vi "fgv_v-linear_func.vi"() -> (3 "velocity_out":dbl)   [LabVIEW 2019]
uses:
  Ctrl/pid-in-params.ctl
  Ctrl/agv_cmd_v.ctl
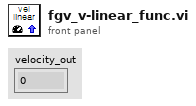
[diagram p1: front panel]
types:
  T1 = typedef "pid-in-params.ctl" = enum16{"read", "write"}
  T2 = cluster{" turn angular speed":dbl, "move linear speed":dbl, "decrease factor linear speed":dbl, "adjust angle margin":dbl}
  T3 = cluster{"deg_agv-lookahead":dbl, "deg_waypoint":dbl, "deg_gap":dbl, "deg_target":dbl, "pid output":dbl, "dis-gap":dbl, "deg_agv-center":dbl}
  T4 = typedef "system_hw.ctl" = cluster{"AGV":enum16{"none", "ERP42", "ERP42mini", "Scout", "Ycar"}, "Lidar 1":enum16{"none", "VLP16", "TIM571", "RPLidar A2", "RPLidar A3"}, "Lidar 2":enum16{"none", "VLP16", "TIM571", "RPLidar A2", "RPLidar A3"}, "GPS":enum16{"none", "F9P", "M8P", "PwrPak7", "19X HVS"}, "Camera":enum16{"none", "C920", "C922", "GT1290C", "MS LifeCam"}, "Joystick":enum16{"none", "joystick"}, "sound":enum16{"none", "speaker"}, "IMU":enum16{"none", "MW-AHRSv1"}}
  T5 = enum16{"none", "ERP42", "ERP42mini", "Scout", "Ycar"}
  T6 = typedef "agv_cmd_v.ctl" = enum16{"write limit", "init stop", "write", "read"}
  T7 = cluster{"limit_linear-v":dbl, "limit_angular-v":dbl}
  T8 = cluster{"Port":refnum<visa-resource-name>, "limits":cluster{"speed limits":cluster{"max":dbl, "min":dbl}, "steer limits":cluster{"max":dbl, "min":dbl}}}
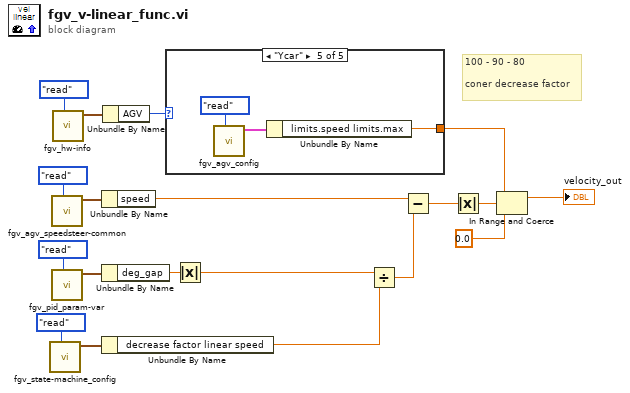
[diagram p0: block diagram]
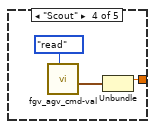
[diagram p5: hidden frame]
diagram:
  # "100 - 90 - 80\n\nconer decrease factor"
  n1 = call "fgv_state-machine_config.vi"("cmd"=enum16{"write", "read"}."read") -> ("Angle cfg out"=w10:T2)  [unwired: 10 in]
  n2 = call "fgv_agv_speedsteer-common.vi"("cmd"=enum16{"init", "read", "write"}."read") -> ("speed-steer out"=w2:cluster{"speed":dbl, "steer":dbl})  [unwired: 9 in, 1 out]
  n3 = call "fgv_pid_param-var.vi"("cmd"=pid-in-params."read") -> ("pid-var_output"=w14:T3)  [unwired: 10 in]
  n4 = call "fgv_hw-info.vi"("cmd"=enum16{"write", "read"}."read") -> ("HW info out"=w5:T4)  [unwired: 10 in]
  n5 = Unbundle By Name(w2) -> ("speed"=w1:dbl)
  n6 = Unbundle By Name(w14) -> ("deg_gap"=w13:dbl)
  n7 = Unbundle By Name(w10) -> ("decrease factor linear speed"=w9:dbl)
  n8 = Unbundle By Name(w5) -> ("AGV"=w4:T5)
  n9 = case shown="\"Ycar\"" w4 {
    tunnel: [_ _ _ w20 w23] -> w17
    frame "none", Default {
    }
    frame "ERP42" {
    }
    frame "ERP42mini" {
    }
    frame "Scout" {
      n10 = call "fgv_agv_cmd-val.vi"("cmd"=agv_cmd_v."read") -> ("limits out"=w21:T7)  [unwired: 9 in, 1 out]
      n11 = Unbundle(w21) -> ("limit_linear-v"=w20:dbl)  [unwired: 1 out]
    }
    frame "Ycar" {
      n12 = call "fgv_agv_config.vi"("cmd"=enum16{"read", "write"}."read") -> ("AGV cfg out"=w24:T8)  [unwired: 9 in, 1 out]
      n13 = Unbundle By Name(w24) -> ("limits.speed limits.max"=w23:dbl)
    }
  }
  n14 = Absolute Value(x=w13) -> (abs(x)=w7:dbl)
  n15 = Divide(x=w7, y=w9) -> (x/y=w15:dbl)
  n16 = Subtract(x=w1, y=w15) -> (x-y=w12:dbl)
  n17 = Absolute Value(x=w12) -> (abs(x)=w8:dbl)
  n18 = In Range and Coerce(upper limit=w17, x=w8, lower limit=0.0 ("하위 리미트")) -> (coerced(x)=→"velocity_out":dbl)  [unwired: 1 out]
